vi "Initialize MeasurementLink Session.vi"(7 "remote connection options":T2, 8 "error in":errorcluster, 9 "initialize session behavior":T1, 10 "resource name":string, 11 "instrument in":refnum<class "Instrument.lvclass">) -> (0 "error out":errorcluster, 2 "session out":variant, 3 "instrument out":refnum<class "Instrument.lvclass">)   [LabVIEW 2020, in "MeasurementLink niDMM.lvlib" / "Instrument.lvclass"]
uses:
  Instrument.lvclass
  MeasurementLink Instrument/IInstrument/Remote Connection Options.ctl
  MeasurementLink Instrument/IInstrument/Initialize Session Behavior.ctl
  Instrument.lvclass/Instrument.ctl
  MeasurementLink Measurement Server/Helpers/Error Strings Global Internal.vi
  MeasurementLink Instrument/IInstrument/IInstrument.lvclass
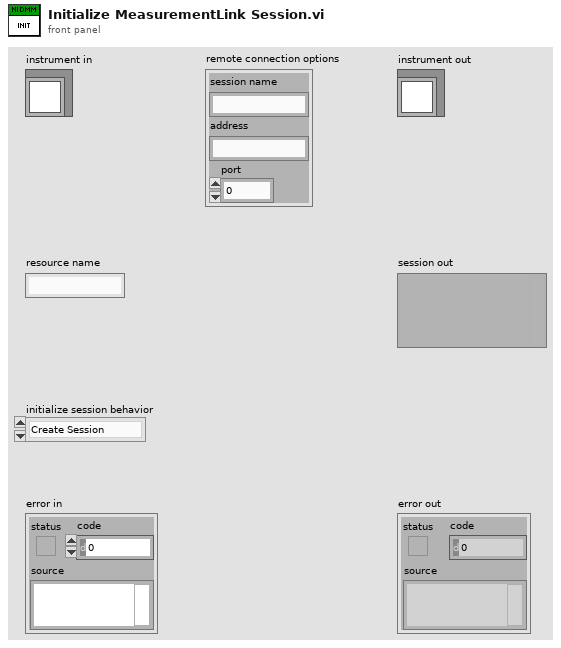
[diagram p1: front panel]
types:
  T1 = typedef "MeasurementLink Instrument.lvlib/IInstrument.lvclass/Initialize Session Behavior.ctl" = enum16{"Create Session", "Attach Session"}
  T2 = typedef "MeasurementLink Instrument.lvlib/IInstrument.lvclass/Remote Connection Options.ctl" = cluster{"session name":string, "address":string, "port":u32}
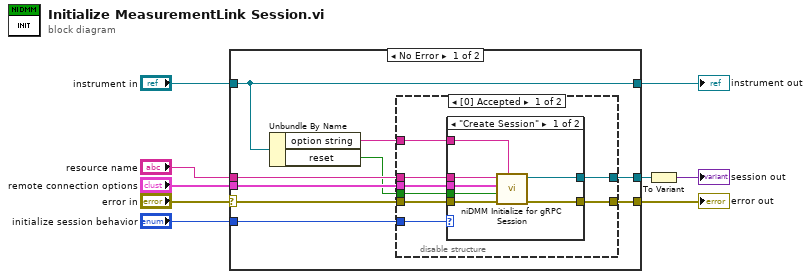
[diagram p0: block diagram]
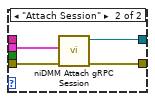
[diagram p2: hidden frame]
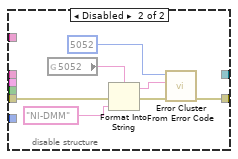
[diagram p3: hidden frame]
diagram:
  n1 = case shown="No Error" "error in" {
    selector: "error in" -> [w15 w45]
    tunnel: [w14 w45] -> w8
    tunnel: "instrument in" -> [w12 w46]
    tunnel: [w12 w46] -> w6
    tunnel: "initialize session behavior" -> [w18 _]
    tunnel: "remote connection options" -> [w17 _]
    tunnel: "resource name" -> [w13 _]
    tunnel: [w16 _] -> w2
    frame No Error {
      n2 = Unbundle By Name(w12) -> ("option string"=w11:string, "reset"=w10:bool)
      n3 = disable-structure shown="[0] Accepted" {
        disable-tunnel: w18 -> [w26 _]
        disable-tunnel: w17 -> [w25 _]
        disable-tunnel: [w24 _] -> w16
        disable-tunnel: w15 -> [w23 w39]
        disable-tunnel: [w22 w38] -> w14
        disable-tunnel: w13 -> [w21 _]
        disable-tunnel: w11 -> [w20 _]
        disable-tunnel: w10 -> [w19 _]
        frame Enabled {
          n4 = case shown="\"Create Session\"" w26 {
            tunnel: w25 -> [w32 w37]
            tunnel: [w31 w36] -> w24
            tunnel: w23 -> [w33 w35]
            tunnel: [w30 w34] -> w22
            tunnel: w21 -> [w29 _]
            tunnel: w20 -> [w28 _]
            tunnel: w19 -> [w27 _]
            frame "Create Session" {
              n5 = call <instrlib>:"niDMM Initialize for gRPC Session.vi"("Option String"=w28, "error in (no error)"=w33, "Reset Device"=w27, "gRPC Options"=w32, "Instrument Descriptor"=w29) -> ("error out"=w30:errorcluster, "instrument handle out"=w31:refnum<k15>)  [unwired: 5 in]
            }
            frame "Attach Session" {
              n6 = call <instrlib>:"niDMM Attach gRPC Session.vi"("error in (no error)"=w35, "gRPC Options"=w37) -> ("error out"=w34:errorcluster, "instrument handle out"=w36:refnum<k15>)  [unwired: 8 in]
            }
          }
        }
        frame Disabled {
          n7 = global read "Error Strings Global Internal.vi" "5052"() -> (w43:string)
          n8 = Format Into String(format string=w43, error in=w39, "NI-DMM") -> (resulting string=w40:string, error out=w41:errorcluster)  [unwired: 1 in]
          n9 = call <vilib>:"Error Cluster From Error Code.vi"("error in (no error)"=w41, "error message (\"\")"=w40, "error code (0)"=5052) -> ("error out"=w38:errorcluster)  [unwired: 6 in]
        }
      }
    }
    frame Error {
    }
  }
  "error out" <- w8
  "instrument out" <- w6
  n10 = To Variant(anything=w2) -> (Variant=→"session out":variant)
